vi "CS_cRIO-PB_MSAC2_DPV1-ReadReq.vi"(0 "FPGA VI Reference":T7, 5 "Slave":i8, 7 "Read data":T5 {"Slot number:" format="%0.0f"; "Communication ref.:" format="%0.0f"}, 11 "Error":errorcluster) -> (4 "FPGA VI Reference out":T7, 6 "Result":T6, 8 "Read response data":T1 {"Error data"."Error decode:" format="%.0x"; "Error data"."Remote address:" format="%0.0f"; "Error data"."Communication ref.:" format="%0.0f"; "Abort data"."Reasoncode:" format="%.0x"; "Abort data"."Instance:" format="%.0x"; "Abort data"."Additional detail:" format="%04x"; "Abort data"."Subnet:" format="%.0x"; "Abort data"."Response SAP:" format="%0.0f"; "Abort data"."Remote address:" format="%0.0f"; "Read data"."Communication ref.:" format="%0.0f"; "Read data"."Data:" format="%.0x"}, 15 "Error out":errorcluster)   [LabVIEW 2013, in "dynamic profibus.lvlib"]
doc: "Reads a DPV1 variable from the DP Slave.\n\nFPGA VI Reference:\nReference of the FPGA VI.\n\nSlave:\nPROFIBUS address of the DPV1 Slave.\n\n\nRead data:\n\nCommunication ref.:\nCommunication reference. Must be identical to that one used with Initiate_req. \n\nSlot number:\nAssigns the slot of the DPV1 data to be read.\n\nIndex:\nAssigns the index of the DPV1 data to be read.\n\nLength:\nAssigns the length of the DPV1 data to be read in bytes.\n\n\nFPGA VI Reference out:\nIs a copy of the FPGA VI Reference .\n\nResult:\nSuccess: The DPV1 Slave responded with a positive confirmation, connection is established.\nAbort: Connection is aborted by DPV1 Master or DPV1 Slave. Check Abort data.\nError: DPV1 Error occured. Check Error data.\n\n\nRead response data:\n\nRead data:\n\nCommunication ref.:\nCommunication reference returned.\n\nRemote address:\nProfibus address of the DPV1 Slave.\n\nLength:\nReceived number of bytes from the DPV1 Slave.\n\nData:\nReceived DPV1 data.\n\n\nAbort data:\n\nThe following values are returned by the Initiate_Req function in case of a negative confirmation (DPV1 Slave refuses connection or DPV1 Master refuses service)\n\nRemote address:\nProfibus address of the DPV1 Slave.\n\nResponse SAP:\nCommunication SAP of the DPV1 Slave.\n\nLocally generated:\nTRUE indicates, that the DPV1 Master refused the connection.\n\nSubnet: Always 0\nInstance: 0 = FDL; 1 = MSAC_C2; 2 = User\n\nReasoncode: \n\nFDL (Instance)\n1 = UE ; 2 = RR ; 3 = RS ; 9 = NR ; 10 = DH ; 11 = LR ; 12 = RDL ; 13 = RDH ; 14 = DS ; 15 = NA \nThe FDL error codes are described in the COMSOFT DP_DPV1_e.pdf document, chapter 5 or in the PROFIBUS standard, FDL Layer.\n\nMSAC_C2 (Instance)\n1 = ABT_SE sequence error; service not allowed in this state\n2 = ABT_FE invalid request PDU received\n3 = ABT_TO timeout of the connection\n4 = ABT_RE invalid response PDU received\n5 = ABT_IV invalid service from USER\n6 = ABT_STO Send_Timeout requested was to small\n7 = ABT_IA invalid additional address information\n8 = ABT_OC waiting for FDL_DATA_REPLY.con\n\nAdditional_Detail:\nThis parameter contains the Send_Timeout received in the RM-REQ-PDU if the instance is MSAC_C2 and the Reason_Code is ABT_STO\n\nUser (Instance)\nManufacturer specific\n\n\nError data:\n\nThe error tab displays DPV1 communication errors.\n\nCommunication ref.:\nThe selected communication reference.\n\nRemote address:\nProfibus address of the DPV1 Slave.\n\nError decode:\n0 to 127 = reserved ; 128 = DPV1 ; 129 to 253 = reserved ; 254 = PROFIBUS FMS ; 255 = HART®\n\nError code 1:\nBit 0 - 3 is the error code, Bit 4 - 7 is the error class\n\nBit 4-7 = 0-9: reserved\n\nBit 4-7 = 10 and Bit 0-3 = 0: read error; 1: write error; 2: module failure; 3 - 7: reserved; 8: version conflict ; 9: feature not supported ; 10 to 15: user specific\n\nBit 4-7 = 11 and Bit 0-3 = 0: invalid index; 1: write length error; 2: invalid slot; 3: type conflict; 4: invalid area; 5: state conflict; 6: access denied; 7: invalid range; 8: invalid parameter; 9: invalid type; 10 to 15: user specific;\n\nBit 4-7 = 12 and Bit 0-3 = 0: read constrain conflict; 1: write constrain conflict; 2: resource busy; 3: resource unavailable; 4 to 7 = reserved; 8 to 15: user specific;\n\nBit 4-7 = 13-15: user specific: \n\nError code 2:\nUser specific\n\n\nError:\nPreceeding error conditions. If an error has already occurred, the VI returns the value of the error in Error out.\n\nError out:\nError: TRUE if an error occurred.\nStatus: Error code\nInfo: Error description"
uses:
  dynamic profibus.lvlib
  fpga reference.ctl
  <vilib>/addons/Comsoft.lib/cRIO PBMS/Examples/SubVIs/CS_PB_DPV1_AbortIndData.ctl
  <vilib>/addons/Comsoft.lib/cRIO PBMS/Examples/SubVIs/CS_PB_DPV1_ErrorData.ctl
  <vilib>/addons/Comsoft.lib/cRIO PBMS/Examples/SubVIs/CS_PB_DPV1_Result.ctl
  <vilib>/addons/Comsoft.lib/cRIO PBMS/Examples/SubVIs/CS_PB_DPV1_ReadConData.ctl
  <vilib>/addons/Comsoft.lib/cRIO PBMS/Examples/SubVIs/CS_PB_DPV1_ReadResData.ctl
  <vilib>/addons/Comsoft.lib/cRIO PBMS/Examples/SubVIs/CS_PB_DPV1_ReadReqData.ctl
panel:
  # "The DPV1 variables of a DP Slave are selected by the parameters Slot number and Index. Refer to the documentation of the DP Slave for a detailed description of all available variables."
  # "- Enter the identical value (1) for Communication ref as used for InitateReq. \n\n- Enter the Slot Number, Index and Length for the DPV1 variable to be read. To enter the DP Slave address is not necessary; this is decoded via the Communication ref parameter, which was assigned as 1 during connection setup.\n\n- Click the DPV1 Read button. After the service is completed, the DPV1 Result has to display Success, what means that DPV1 data has been successfully read from the DP Slave.\n\nIf the Result does not display Success, check the Abort and Error section. See Context Help for detailed description of error checking."
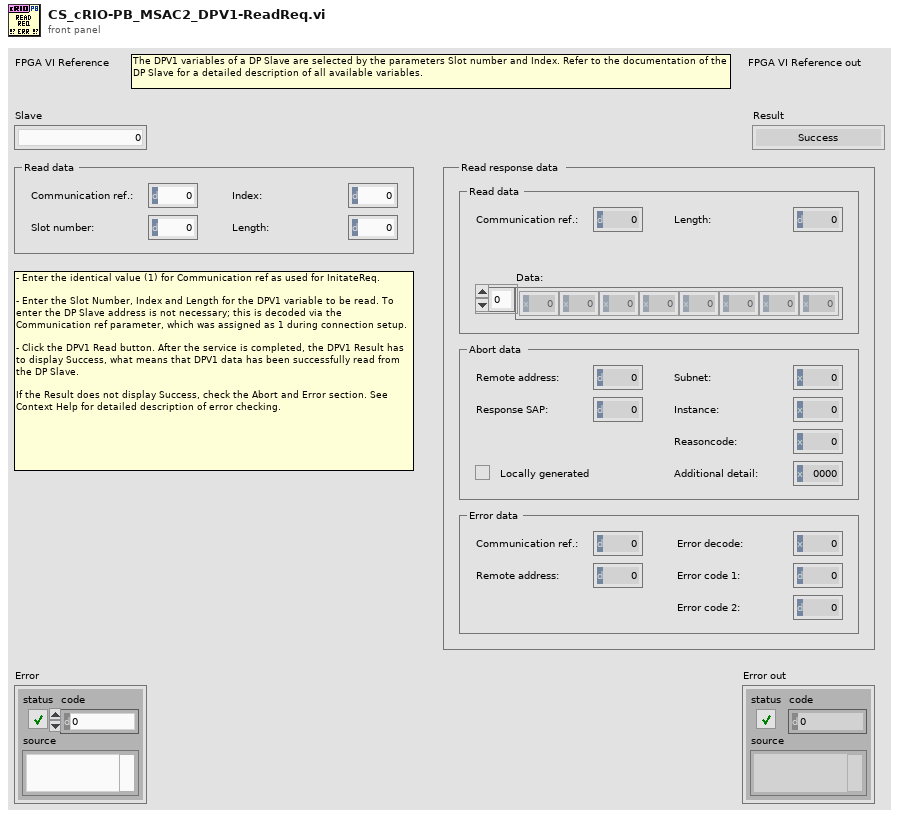
[diagram p1: front panel]
types:
  T1 = typedef "CS_PB_DPV1_ReadResData.ctl" = cluster{"Read data":T2, "Abort data":T3, "Error data":T4}
  T2 = typedef "CS_PB_DPV1_ReadConData.ctl" = cluster{"Communication ref.:":u8, "Length:":u8, "Data:":u8[]}
  T3 = typedef "CS_PB_DPV1_AbortIndData.ctl" = cluster{"Remote address:":u8, "Response SAP:":u8, "Locally generated":bool, "Subnet:":u8, "Instance:":u8, "Reasoncode:":u8, "Additional detail:":u16}
  T4 = typedef "CS_PB_DPV1_ErrorData.ctl" = cluster{"Communication ref.:":u8, "Remote address:":u8, "Error decode:":u8, "Error code 1:":u8, "Error code 2:":u8}
  T5 = typedef "CS_PB_DPV1_ReadReqData.ctl" = cluster{"Communication ref.:":u8, "Slot number:":u8, "Index:":u8, "Length:":u8}
  T6 = typedef "CS_PB_DPV1_Result.ctl" = enum16{"Success", "Abort", "Error"}
  T7 = typedef "dynamic profibus.lvlib/fpga reference.ctl" = refnum<k20>
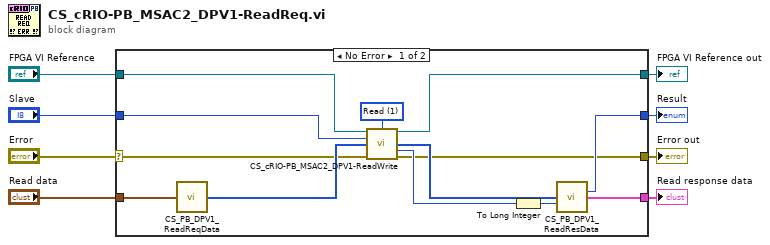
[diagram p0: block diagram]
diagram:
  n1 = case shown="No Error" "Error" {
    selector: "Error" -> [w13 w22]
    tunnel: "Slave" -> [w9 _]
    tunnel: "FPGA VI Reference" -> [w11 w23]
    tunnel: [w12 w23] -> w8
    tunnel: [w14 w22] -> w5
    tunnel: [w15 _] -> w6
    tunnel: [w18 _] -> w4
    tunnel: "Read data" -> [w17 _]
    frame No Error {
      w10 = i8 1 items=["Initiate", "Read", "Write", "Abort"] ("DPV1-Service")
      n2 = call <vilib>:"CS_PB_DPV1_ReadReqData.vi"("Read data"=w17) -> ("Request data"=w20:u8[])  [unwired: 14 in]
      n3 = call "CS_cRIO-PB_MSAC2_DPV1-ReadWrite.vi"("FPGA VI Reference"=w11, "DPV1-Service"=w10, "Slave"=w9, "Data"=w20, "Error"=w13) -> ("FPGA VI Reference out"=w12:T7, "Data out"=w19:u8[], "Status"=w21:u8, "Error out"=w14:errorcluster)  [unwired: 7 in]
      n4 = To Long Integer(number=w21) -> (32bit integer=w16:i32)
      n5 = call <vilib>:"CS_PB_DPV1_ReadResData.vi"("Response data"=w19, "Status"=w16) -> ("Result"=w18:T6, "Read response data"=w15:T1)  [unwired: 12 in]
    }
    frame Error {
    }
  }
  "Error out" <- w5
  "FPGA VI Reference out" <- w8
  "Result" <- w4
  "Read response data" <- w6
